vi "Append New Styled Paragraph.vi"(8 "error in (no error)":errorcluster, 9 "Type":T1(ring), 10 "Paragraph.Text":string, 11 "xwpfDocument in":refnum<class "xwpfDocument.lvclass">) -> (0 "error out":errorcluster, 3 "xwpfDocument out":refnum<class "xwpfDocument.lvclass">)   [LabVIEW 2017, in "Word_Specific.lvlib" / "xwpfDocument.lvclass"]
uses:
  xwpfDocument.lvclass
  xwpfDocument.lvclass/xwpfDocument.ctl
  C:/Program Files (x86)/National Instruments/LabVIEW 2017/vi.lib/BenjaminR/LabVIEW NPOI/lib/NPOI 2.1.1/NPOI.OOXML.dll
  Program Files (x86)/National Instruments/LabVIEW 2017/vi.lib/BenjaminR/LabVIEW NPOI/lib/NPOI 2.1.1/NPOI.OOXML.dll
  xwpfParagraph/xwpfParagraph.lvclass
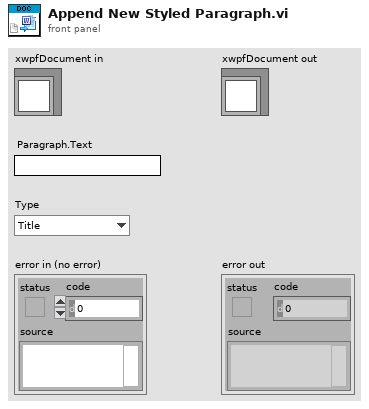
[diagram p1: front panel]
types:
  T1 = enum16{"Title", "Heading 1", "Heading 2", "Heading 3", "Normal", "Figure", "Page Break"}
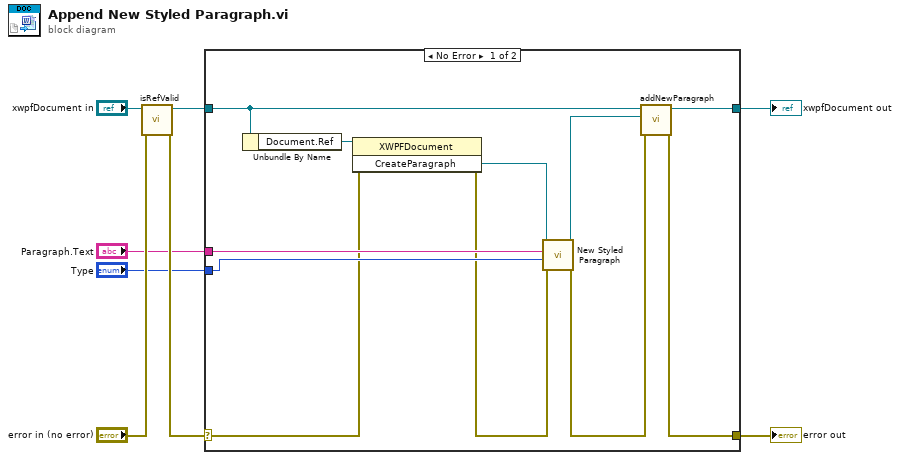
[diagram p0: block diagram]
diagram:
  n1 = call-dynamic "isRefValid.vi"("error in (no error)"="error in (no error)", "xwpfDocument in"="xwpfDocument in") -> ("error out"=w3:errorcluster, "xwpfDocument out"=w5:refnum<class "xwpfDocument.lvclass">)  [unwired: 8 in]
  n2 = case shown="No Error" w3 {
    selector: w3 -> [w9 w21]
    tunnel: [w16 w21] -> w8
    tunnel: [w19 w20] -> w6
    tunnel: w5 -> [w13 w20]
    tunnel: "Paragraph.Text" -> [w15 _]
    tunnel: "Type" -> [w14 _]
    frame No Error {
      n3 = Unbundle By Name(w13) -> ("Document.Ref"=w10:refnum<k24>)
      n4 = invoke class="XWPFDocument" method="CreateParagraph"(reference=w10, error in=w9) -> (error out=w12:errorcluster, "CreateParagraph"=w11:refnum<k24>)  [unwired: 1 in, 1 out]
      n5 = call "New Styled Paragraph.vi"("error in (no error)"=w12, "Type"=w14, "Paragraph.Text"=w15, "Paragraph.Ref"=w11) -> ("error out"=w17:errorcluster, "xwpfParagraph out"=w18:refnum<class "xwpfParagraph.lvclass">)  [unwired: 6 in]
      n6 = call "addNewParagraph.vi"("error in (no error)"=w17, "New Paragraph"=w18, "xwpfDocument in"=w13) -> ("error out"=w16:errorcluster, "xwpfDocument out"=w19:refnum<class "xwpfDocument.lvclass">)  [unwired: 7 in]
    }
    frame Error {
    }
  }
  "error out" <- w8
  "xwpfDocument out" <- w6
